vi "Resolve DB Bin File Name and Path.vi"(8 "error in":errorcluster, 10 "Path to Tools":path, 11 "DB XML File":path) -> (0 "error out":errorcluster, 1 "SysExec":string, 2 "Converted File Destination":path, 3 "Converted File Source":path)   [LabVIEW 2013, in "AIT 1553 Custom Device.lvlib"]
uses:
  AIT 1553 Custom Device.lvlib
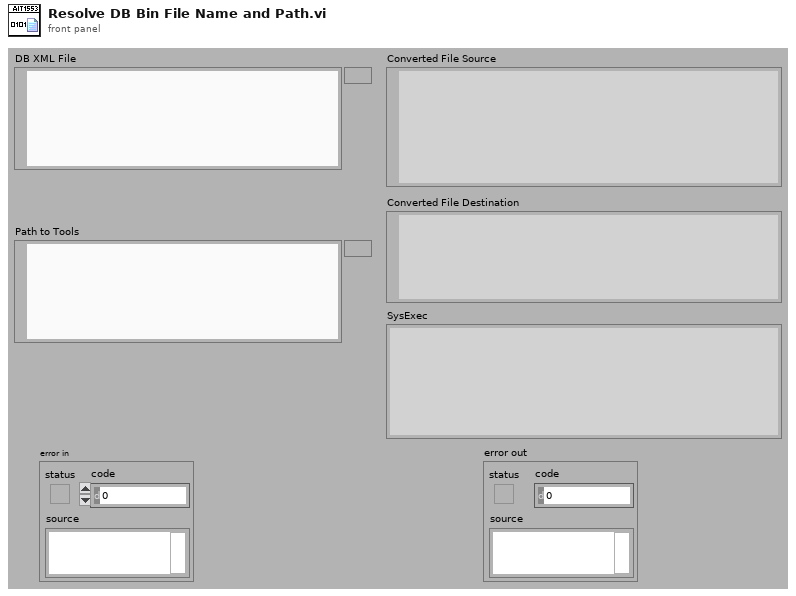
[diagram p1: front panel]
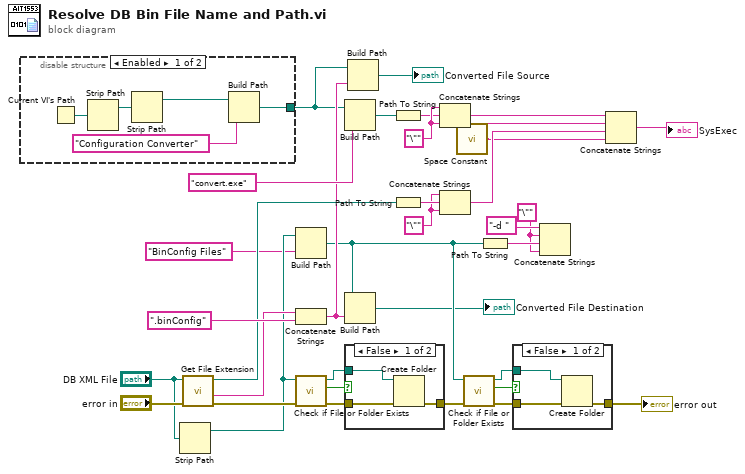
[diagram p0: block diagram]
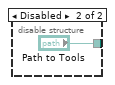
[diagram p3: hidden frame]
diagram:
  w12 = "\"" ("string")
  w27 = "\"" ("string")
  w31 = "\"" ("string")
  n1 = disable-structure shown="Enabled" {
    disable-tunnel: [w36 "Path to Tools"] -> w9
    frame Enabled {
      n2 = Current VI's Path() -> (path=w39:path)
      n3 = Strip Path(path=w39) -> (stripped path=w38:path)  [unwired: 1 out]
      n4 = Strip Path(path=w38) -> (stripped path=w37:path)  [unwired: 1 out]
      n5 = Build Path(base path=w37, name or relative path="Configuration Converter") -> (appended path=w36:path)
    }
    frame Disabled {
    }
  }
  n6 = Strip Path(path="DB XML File") -> (stripped path=w16:path)  [unwired: 1 out]
  n7 = call <vilib>:"Get File Extension.vi"("error in (no error)"="error in", "file"="DB XML File") -> ("error out"=w22:errorcluster, "filename without extension"=w33:string, "dup file"=w23:path)  [unwired: 6 in, 1 out]
  n8 = Build Path(base path=w16, name or relative path="BinConfig Files" ("string")) -> (appended path=w4:path)
  n9 = Concatenate Strings(w33, ".binConfig" ("string")) -> (w10:string)
  n10 = call <vilib>:"Check if File or Folder Exists.vi"("error in (no error)"=w22, "path"=w16) -> ("error out"=w20:errorcluster, "file or folder exists?"=w21:bool, "dup path"=w19:path)  [unwired: 7 in]
  n11 = Build Path(base path=w9, name or relative path="convert.exe") -> (appended path=w30:path)
  n12 = Build Path(base path=w4, name or relative path=w10) -> (appended path=→"Converted File Destination":path)
  n13 = case shown="False" w21 {
    tunnel: [w41 w44] -> w5
    tunnel: w20 -> [w43 w44]
    tunnel: w19 -> [w42 _]
    frame False {
      n14 = Create Folder(path (use dialog)=w42, error in=w43) -> (error out=w41:errorcluster)  [unwired: 1 in, 2 out]
    }
    frame True {
    }
  }
  n15 = Build Path(base path=w9, name or relative path=w10) -> (appended path=→"Converted File Source":path)
  n16 = Path To String(path=w30) -> (string=w29:string)
  n17 = Path To String(path=w23) -> (string=w28:string)
  n18 = Concatenate Strings(w31, w29, w31) -> (w24:string)
  n19 = Concatenate Strings(w27, w28, w27) -> (w26:string)
  n20 = call <vilib>:"Space Constant.vi"() -> ("String"=w11:string)
  n21 = call <vilib>:"Check if File or Folder Exists.vi"("error in (no error)"=w5, "path"=w4) -> ("error out"=w7:errorcluster, "file or folder exists?"=w6:bool, "dup path"=w8:path)  [unwired: 7 in]
  n22 = Path To String(path=w4) -> (string=w13:string)
  n23 = case shown="False" w6 {
    tunnel: [w45 w48] -> w3
    tunnel: w7 -> [w47 w48]
    tunnel: w8 -> [w46 _]
    frame False {
      n24 = Create Folder(path (use dialog)=w46, error in=w47) -> (error out=w45:errorcluster)  [unwired: 1 in, 2 out]
    }
    frame True {
    }
  }
  "error out" <- w3
  n25 = Concatenate Strings("-d " ("string"), w12, w13, w12) -> ()  [unwired: 1 out]
  n26 = Concatenate Strings(w24, w11, w26, w11) -> (→"SysExec":string)
